vi "Initialize.vi"(8 "error in (no error)":errorcluster, 11 "dmp_sample_rate":i32=100) -> (0 "error out":errorcluster, 1 "IMU Data":T1, 2 "Event Registration Refnum":refnum<event-registration>, 3 "IMU Event":refnum<user-event>)   [LabVIEW 2014]
uses:
  Interrupt/LV/Interrupt.lvlib
  <userlib>/UCSD Robotics Lab/Robotics-Cape/LV/libroboticscape.lvlib
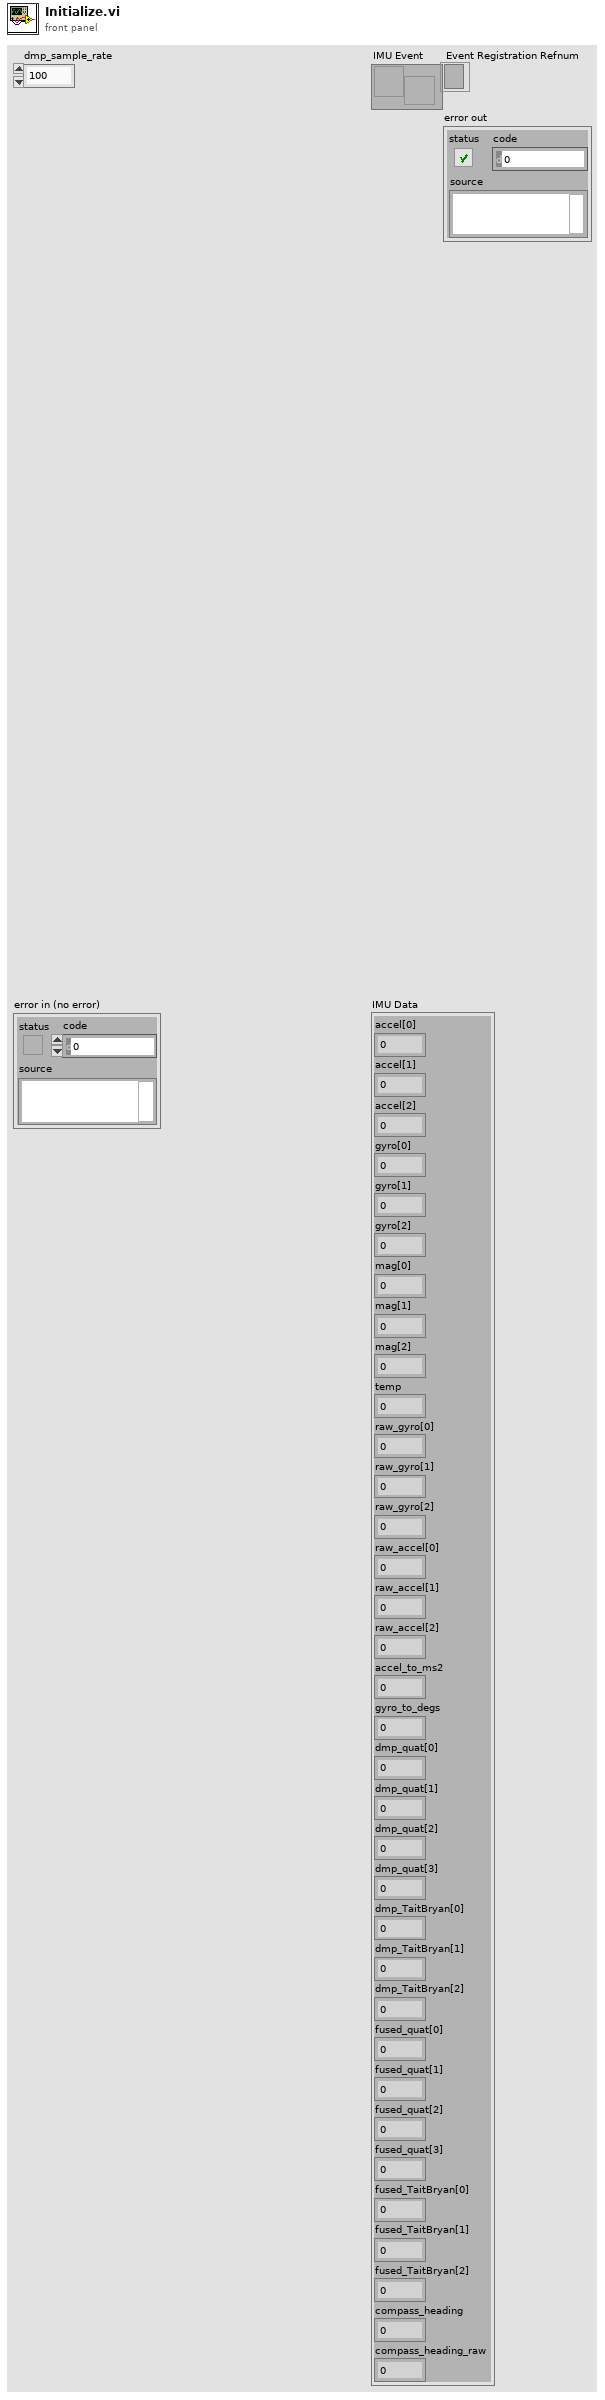
[diagram p1: front panel]
types:
  T1 = cluster{"accel[0]":sgl, "accel[1]":sgl, "accel[2]":sgl, "gyro[0]":sgl, "gyro[1]":sgl, "gyro[2]":sgl, "mag[0]":sgl, "mag[1]":sgl, "mag[2]":sgl, "temp":sgl, "raw_gyro[0]":i16, "raw_gyro[1]":i16, "raw_gyro[2]":i16, "raw_accel[0]":i16, "raw_accel[1]":i16, "raw_accel[2]":i16, "accel_to_ms2":sgl, "gyro_to_degs":sgl, "dmp_quat[0]":sgl, "dmp_quat[1]":sgl, "dmp_quat[2]":sgl, "dmp_quat[3]":sgl, "dmp_TaitBryan[0]":sgl, "dmp_TaitBryan[1]":sgl, "dmp_TaitBryan[2]":sgl, "fused_quat[0]":sgl, "fused_quat[1]":sgl, "fused_quat[2]":sgl, "fused_quat[3]":sgl, "fused_TaitBryan[0]":sgl, "fused_TaitBryan[1]":sgl, "fused_TaitBryan[2]":sgl, "compass_heading":sgl, "compass_heading_raw":sgl}
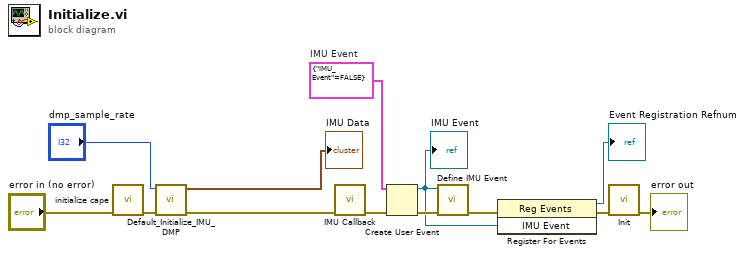
[diagram p0: block diagram]
diagram:
  w12 = cluster{"IMU_Event":bool} {"IMU_Event"=FALSE}  # IMU Event
  n1 = call <userlib>:"initialize cape.vi"("error in (no error)"="error in (no error)") -> ("error out"=w10:errorcluster)  [unwired: 9 in, 1 out]
  n2 = call "Default_Initialize_IMU_DMP.vi"("error in (no error)"=w10, "dmp_sample_rate"="dmp_sample_rate") -> ("error out"=w9:errorcluster, "Data Out"=→"IMU Data":T1)  [unwired: 7 in]
  n3 = call "IMU Callback.vi"("error in (no error)"=w9) -> ("error out"=w8:errorcluster)  [unwired: 9 in, 1 out]
  n4 = Create User Event(user event datatype=w12, error in=w8) -> (user event=w5:refnum<user-event>, error out=w7:errorcluster)
  "IMU Event" <- w5
  n5 = call "Define IMU Event.vi"("error in (no error)"=w7, "user event out"=w5) -> ("error out"=w6:errorcluster)  [unwired: 8 in, 1 out]
  n6 = register-events(error in=w6, w5) -> (reference out=→"Event Registration Refnum":refnum<event-registration>, error out=w3:errorcluster)  [unwired: 1 in]
  n7 = call "Init.vi"("error in (no error)"=w3) -> ("error out"=→"error out":errorcluster)  [unwired: 9 in, 1 out]
